vi "Read Position.vi"(8 "error in (no error)":errorcluster, 11 "AxisCard in":refnum<class "AxisCard.lvclass">) -> (0 "error out":errorcluster, 2 "Position":dbl, 3 "AxisCard out":refnum<class "AxisCard.lvclass">)   [LabVIEW 2019, in "AxisCard.lvclass"]
uses:
  AxisCard.lvclass
  AxisCard.lvclass/AxisCard.ctl
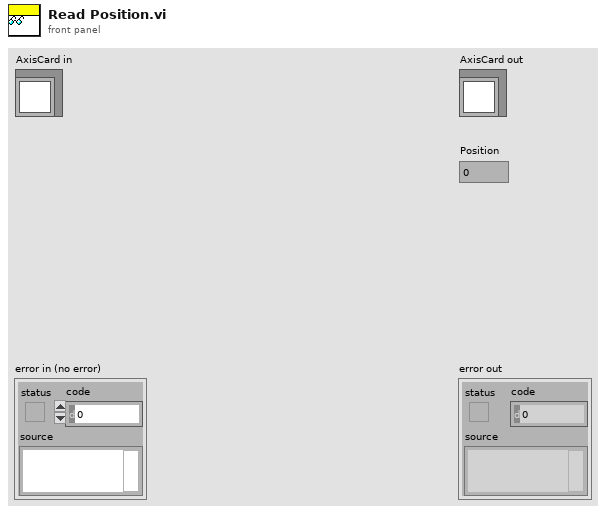
[diagram p1: front panel]
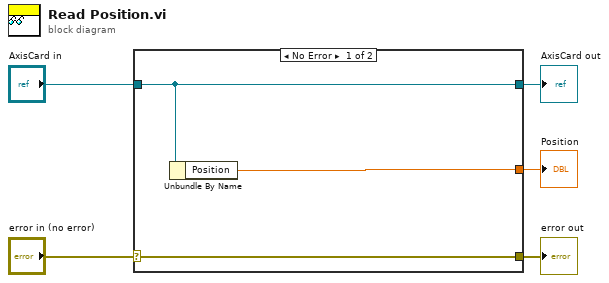
[diagram p0: block diagram]
diagram:
  n1 = case shown="No Error" "error in (no error)" {
    selector: "error in (no error)" -> [w8 w9]
    tunnel: [w8 w9] -> w4
    tunnel: [w7 w10] -> w2
    tunnel: "AxisCard in" -> [w7 w10]
    tunnel: [w6 _] -> w1
    frame No Error {
      n2 = Unbundle By Name(w7) -> ("Position"=w6:dbl)
    }
    frame Error {
    }
  }
  "error out" <- w4
  "AxisCard out" <- w2
  "Position" <- w1
